vi "(SubVI)System Command_Find Auto I2C ID.vi"(8 "error in (no error)":errorcluster caption="에러 입력(에러 없음)") -> (0 "error out":errorcluster caption="에러 출력", 2 "Count":u8, 3 "ID":u8[](array[numeric]))   [LabVIEW 2020]
uses:
  Serial/Controls/(Ctrl)Serial_Write Read Option.ctl
  Serial/Instance VIs/(SubVI)Serial_Write-Read.vi
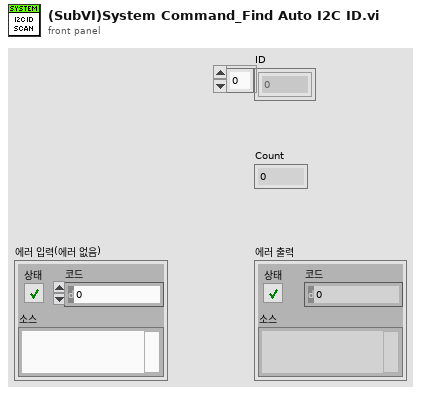
[diagram p1: front panel]
types:
  T1 = typedef "(Ctrl)Serial_Write Read Option.ctl" = cluster{"Echo Request":bool, "Header Verification":bool, "Checksum Verification":bool, "User Code Verifiaction":bool}
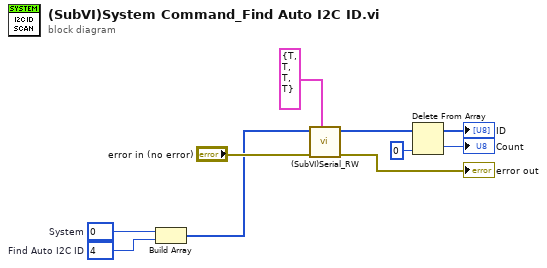
[diagram p0: block diagram]
diagram:
  w8 = u8 4  # Find Auto I2C ID
  w9 = u8 0  # System
  n1 = Build Array(w9, w8) -> (w4:u8[])
  n2 = call-poly "(SubVI)Serial_RW.vi"("Option"=T1 {"Echo Request"=TRUE, "Header Verification"=TRUE, "Checksum Verification"=TRUE, "User Code Verifiaction"=TRUE}, "error in (no error)"="error in (no error)", "Data to Write"=w4) -> ("error out"=→"error out":errorcluster, "Read Data"=w7:u8[])  [unwired: 6 in, 1 out]
  n3 = Delete From Array(array=w7, index=0 ("인덱스")) -> (deleted portion=→"Count":u8, array with subset deleted=→"ID":u8[])  [unwired: 1 in]
